vi "CHS_TRAJECTORY_EXECUTE_ABS.vi"(6 "Pass_Through_Time":dbl=-1.0 format="%33.4f", 8 "Init":bool, 11 "TrajectoryName":string) -> (1 "Complete":bool, 2 "AtReference":bool, 3 "Chassis Velocity Target SI":T1 {"vOmega" format="%10.3f"; "vY" format="%10.3f"; "vX" format="%10.3f"})   [LabVIEW 2019]
uses:
  CHS_TRAJECTORY_GLOBALS.vi
  <vilib>/Rock Robotics/WPI/ThirdParty/JAS_Junk/TrajLib/Trajectory_Library.lvlib
  <vilib>/Rock Robotics/WPI/ThirdParty/ChoreoLib/ChoreoLib.lvlib
  <vilib>/Rock Robotics/WPI/ThirdParty/JAS_Junk/TrajLib/TypeDef/CHASSIS_SPEEDS.ctl
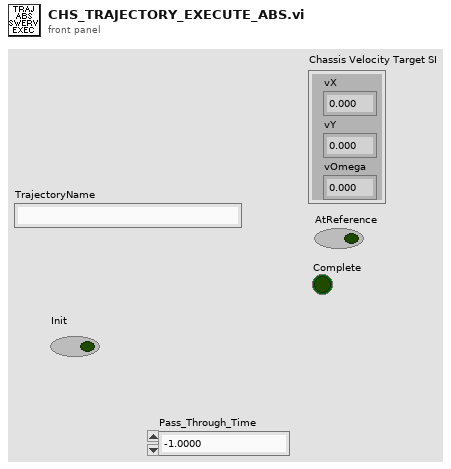
[diagram p1: front panel]
types:
  T1 = typedef "Trajectory_Library.lvlib/CHASSIS_SPEEDS.ctl" = cluster{"vX":dbl, "vY":dbl, "vOmega":dbl}
  T2 = typedef "Trajectory_Library.lvlib/PID_ADV_LIMITS.ctl" = cluster{"MaxInput":dbl, "MinInput":dbl, "Continuous":bool, "MaxOutput":dbl, "MinOutput":dbl}
  T3 = typedef "Trajectory_Library.lvlib/PID_ADV_TUNING.ctl" = cluster{"Kf":dbl, "Kp":dbl, "Ki":dbl, "Kd":dbl, "MaximumIntegral":dbl, "MinimumIntegral":dbl, "Filter Derivative":bool, "IntegralZone":dbl}
  T4 = typedef "Trajectory_Library.lvlib/POSE2D.ctl" = cluster{"TRANSLATION":T5, "ROTATION":T6}
  T5 = typedef "Trajectory_Library.lvlib/TRANSLATION2D.ctl" = cluster{"X":dbl, "Y":dbl}
  T6 = typedef "Trajectory_Library.lvlib/ROTATION2D.ctl" = cluster{"VALUE":dbl, "COS":dbl, "SIN":dbl}
  T7 = typedef "ChoreoLib.lvlib/ChoreoSwerveControlConfig.ctl" = cluster{"X_Adv PID Tuning":T3, "X_Adv PID Limits":T2, "Y_Adv PID Tuning":T3, "Y_Adv PID Limits":T2, "Rot_Adv PID Tuning":T3, "Rot_Adv PID Limits":T2, "X Y Pos Tolerance M":dbl, "Rot Tolerance Deg":dbl, "X Y Vel Tolerance M/S":dbl, "Rot Vel Tolerance Deg/S":dbl}
  T8 = cluster{"X Pos Err M":dbl, "X Vel Err M/S":dbl, "Y Pos Err M":dbl, "Y Vel Err M/S":dbl, "Rot Pos Err Deg":dbl, "Rot Vel Err Deg/Sec":dbl}
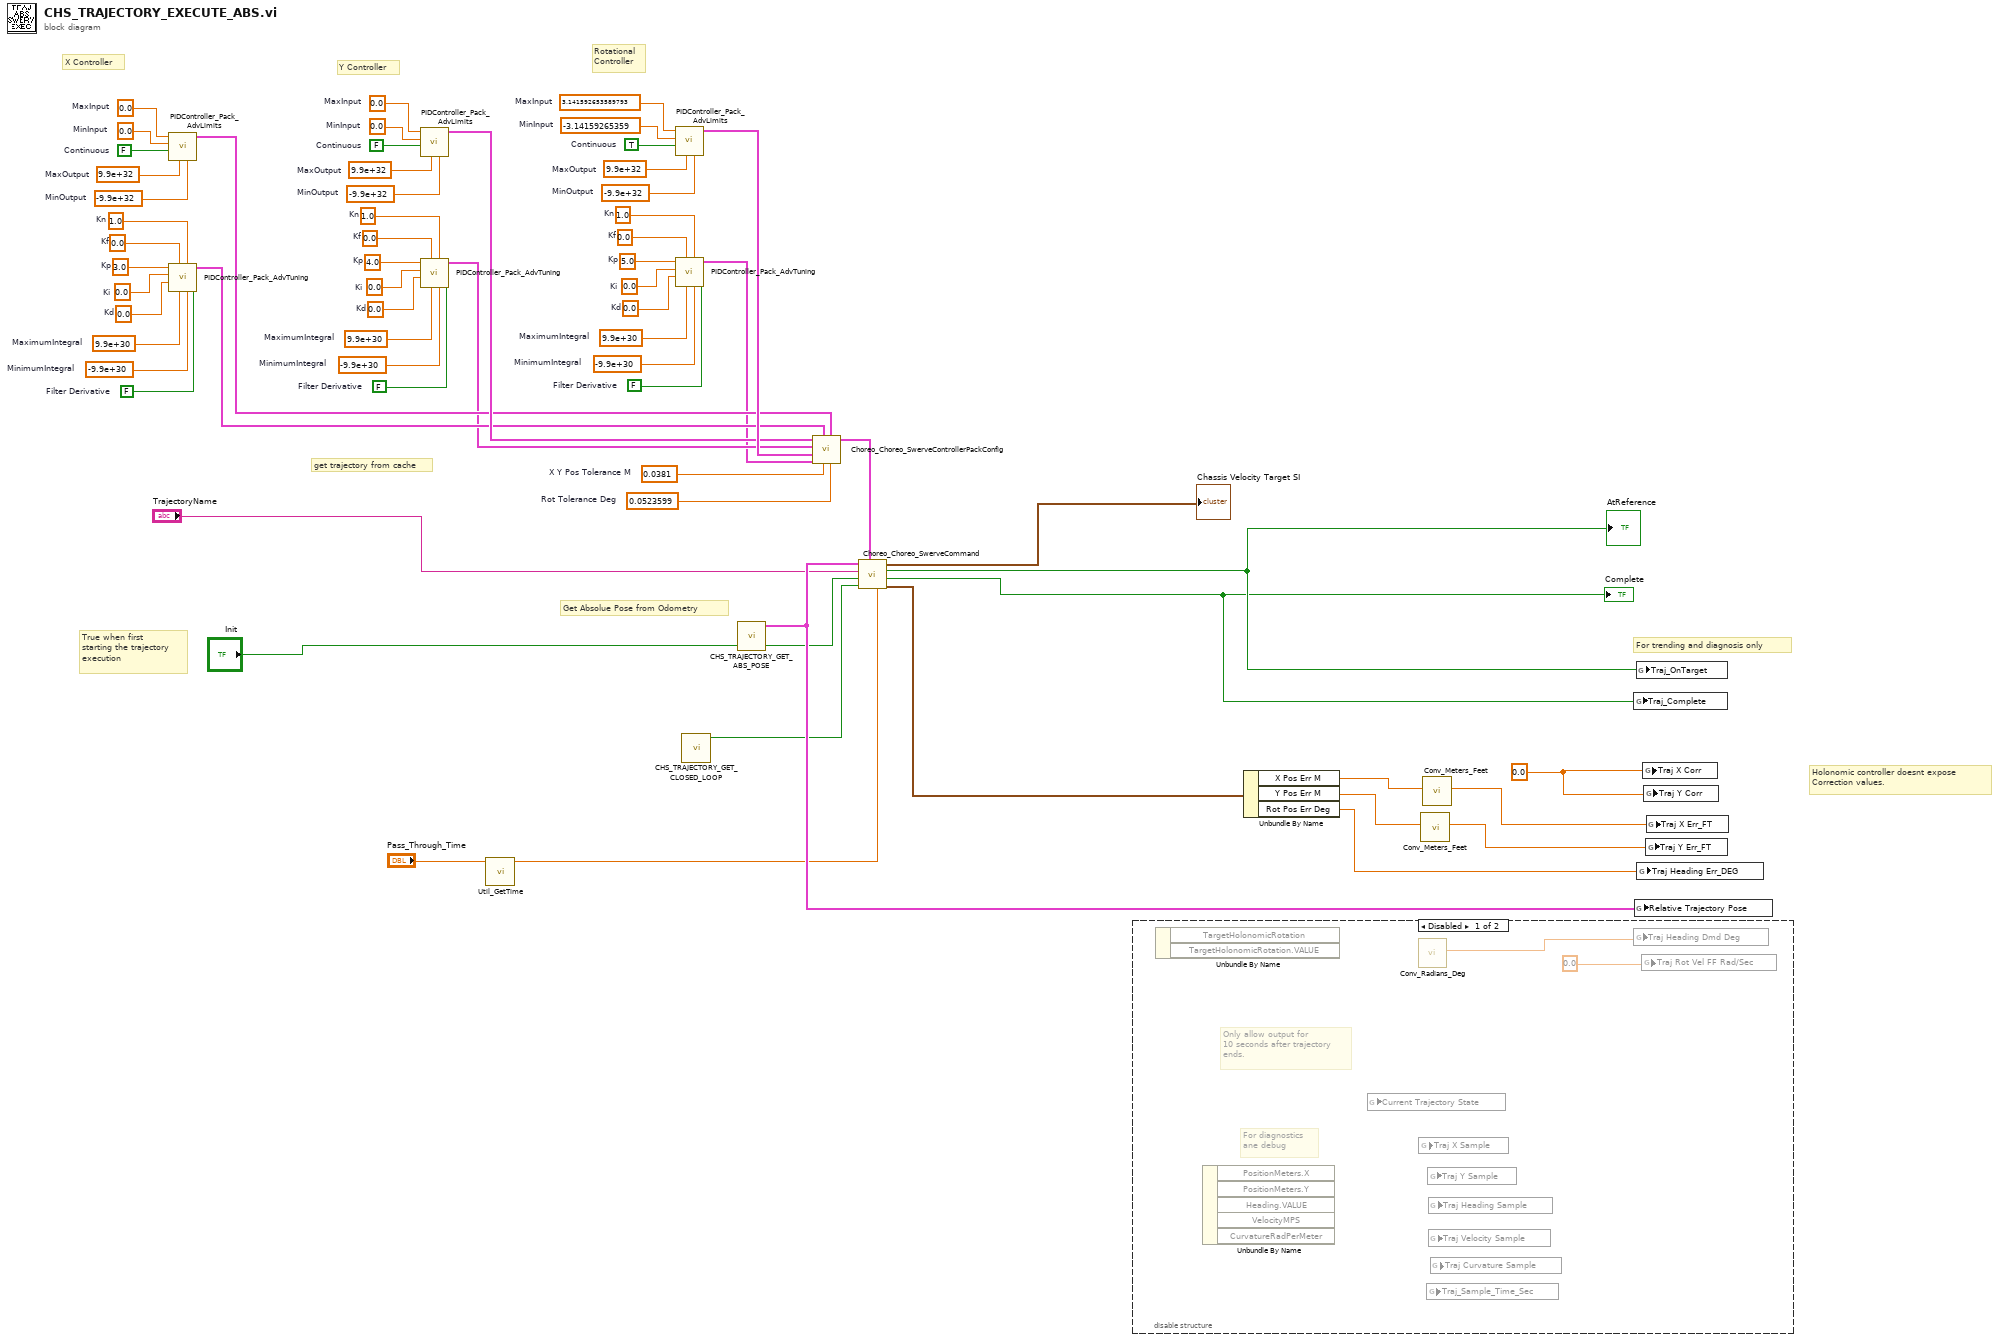
[diagram p0: block diagram]
diagram:
  w9 = 0.0 ("Y Corr")
  w64 = 0.0523599  # Rot Tolerance Deg
  w63 = 0.0381  # X Y Pos Tolerance M
  w44 = 1.0  # Kn
  w45 = 5.0  # Kp
  w46 = 0.0  # Ki
  w47 = 0.0  # Kd
  w48 = 0.0  # Kf
  w49 = 9.9e+30  # MaximumIntegral
  w50 = -9.9e+30  # MinimumIntegral
  w51 = FALSE  # Filter Derivative
  w53 = -3.14159265359  # MinInput
  w54 = TRUE  # Continuous
  w55 = 9.9e+32  # MaxOutput
  w52 = -9.9e+32  # MinOutput
  w56 = 3.141592653589793  # MaxInput
  w31 = 1.0  # Kn
  w32 = 4.0  # Kp
  w33 = 0.0  # Ki
  w34 = 0.0  # Kd
  w35 = 0.0  # Kf
  w36 = 9.9e+30  # MaximumIntegral
  w37 = -9.9e+30  # MinimumIntegral
  w38 = FALSE  # Filter Derivative
  w40 = 0.0  # MinInput
  w41 = FALSE  # Continuous
  w42 = 9.9e+32  # MaxOutput
  w39 = -9.9e+32  # MinOutput
  w43 = 0.0  # MaxInput
  w18 = 1.0  # Kn
  w19 = 3.0  # Kp
  w20 = 0.0  # Ki
  w21 = 0.0  # Kd
  w22 = 0.0  # Kf
  w23 = 9.9e+30  # MaximumIntegral
  w24 = -9.9e+30  # MinimumIntegral
  w25 = FALSE  # Filter Derivative
  w27 = 0.0  # MinInput
  w28 = FALSE  # Continuous
  w29 = 9.9e+32  # MaxOutput
  w26 = -9.9e+32  # MinOutput
  w30 = 0.0  # MaxInput
  # "get trajectory from cache"
  # "Rotational\nController"
  # "Y Controller"
  # "X Controller"
  # "True when first\nstarting the trajectory\nexecution"
  # "Holonomic controller doesnt expose\nCorrection values."
  # "For trending and diagnosis only"
  # "Get Absolue Pose from Odometry"
  n1 = call <vilib>:"PIDController_Pack_AdvLimits.vi"("MinOutput"=w26, "MaxOutput"=w29, "Continuous"=w28, "MinInput"=w27, "MaxInput"=w30) -> ("Adv PID Limits"=w60:T2)  [unwired: 6 in]
  n2 = call <vilib>:"PIDController_Pack_AdvTuning.vi"("Filter Derivative"=w25, "MinimumIntegral"=w24, "Kn"=w18, "MaximumIntegral"=w23, "Kf"=w22, "Kd"=w21, "Ki"=w20, "Kp"=w19) -> ("Adv PID Tuning"=w59:T3)  [unwired: 3 in]
  n3 = call <vilib>:"PIDController_Pack_AdvLimits.vi"("MinOutput"=w39, "MaxOutput"=w42, "Continuous"=w41, "MinInput"=w40, "MaxInput"=w43) -> ("Adv PID Limits"=w61:T2)  [unwired: 6 in]
  n4 = call <vilib>:"PIDController_Pack_AdvTuning.vi"("Filter Derivative"=w38, "MinimumIntegral"=w37, "Kn"=w31, "MaximumIntegral"=w36, "Kf"=w35, "Kd"=w34, "Ki"=w33, "Kp"=w32) -> ("Adv PID Tuning"=w58:T3)  [unwired: 3 in]
  n5 = call <vilib>:"Util_GetTime.vi"("Pass_Through_Time"="Pass_Through_Time") -> ("FPGA_Time_Seconds"=w10:dbl)  [unwired: 8 in, 2 out]
  n6 = call <vilib>:"PIDController_Pack_AdvLimits.vi"("MinOutput"=w52, "MaxOutput"=w55, "Continuous"=w54, "MinInput"=w53, "MaxInput"=w56) -> ("Adv PID Limits"=w62:T2)  [unwired: 6 in]
  n7 = call <vilib>:"PIDController_Pack_AdvTuning.vi"("Filter Derivative"=w51, "MinimumIntegral"=w50, "Kn"=w44, "MaximumIntegral"=w49, "Kf"=w48, "Kd"=w47, "Ki"=w46, "Kp"=w45) -> ("Adv PID Tuning"=w57:T3)  [unwired: 3 in]
  n8 = call "CHS_TRAJECTORY_GET_CLOSED_LOOP.vi"() -> ("AUTO_CLOSED_LOOP"=w15:bool)  [unwired: 11 in]
  n9 = call "CHS_TRAJECTORY_GET_ABS_POSE.vi"() -> ("Absolute Odometry Pose"=w16:T4)  [unwired: 11 in]
  n10 = call <vilib>:"Choreo_Choreo_SwerveControllerPackConfig.vi"("Rot Tolerance Deg"=w64, "X_Adv PID Limits"=w60, "X Y Pos Tolerance M"=w63, "X_Adv PID Tuning"=w59, "Rot_Adv PID Tuning"=w57, "Rot_Adv PID Limits"=w62, "Y_Adv PID Tuning"=w58, "Y_Adv PID Limits"=w61) -> ("ChoreoSwerveControlConfig"=w17:T7)  [unwired: 3 in]
  n11 = call <vilib>:"Choreo_Choreo_SwerveCommand.vi"("Pass_Through_Time"=w10, "ChoreoSwerveControlConfig"=w17, "Auto"=w15, "Initialize"="Init", "TrajectoryName"="TrajectoryName", "Current Position"=w16) -> ("Ctrl Info"=w6:T8, "Complete"=w12:bool, "On Target"=w13:bool, "Chassis Speed Dmd"=→"Chassis Velocity Target SI":T1)  [unwired: 2 in]
  "AtReference" <- w13
  "Complete" <- w12
  n12 = disable-structure shown="Disabled" {
    frame Disabled {
      # "For diagnostics\nane debug"
      # "Only allow output for\n10 seconds after trajectory\nends."
      n13 = Unbundle By Name() -> ()  [unwired: 1 in, 2 out]
      n14 = Unbundle By Name() -> ()  [unwired: 1 in, 5 out]
      n15 = global read "CHS_TRAJECTORY_GLOBALS.vi" "Current Trajectory State"() -> ()  [unwired: 1 in]
      n16 = call <vilib>:"Conv_Radians_Deg.vi"() -> ("Degrees"=w65:dbl)  [unwired: 11 in]
      n17 = global read "CHS_TRAJECTORY_GLOBALS.vi" "Traj X Sample"() -> ()  [unwired: 1 in]
      n18 = global read "CHS_TRAJECTORY_GLOBALS.vi" "Traj_Sample_Time_Sec"() -> ()  [unwired: 1 in]
      n19 = global read "CHS_TRAJECTORY_GLOBALS.vi" "Traj Y Sample"() -> ()  [unwired: 1 in]
      n20 = global read "CHS_TRAJECTORY_GLOBALS.vi" "Traj Heading Sample"() -> ()  [unwired: 1 in]
      n21 = global read "CHS_TRAJECTORY_GLOBALS.vi" "Traj Velocity Sample"() -> ()  [unwired: 1 in]
      n22 = global read "CHS_TRAJECTORY_GLOBALS.vi" "Traj Curvature Sample"() -> ()  [unwired: 1 in]
      n23 = global write "CHS_TRAJECTORY_GLOBALS.vi" "Traj Heading Dmd Deg"(w65) -> ()
      n24 = global write "CHS_TRAJECTORY_GLOBALS.vi" "Traj Rot Vel FF Rad/Sec"(0.0 ("Traj Heading Dmd Deg")) -> ()
    }
    frame Enabled {
    }
  }
  n25 = Unbundle By Name(w6) -> ("X Pos Err M"=w5:dbl, "Y Pos Err M"=w4:dbl, "Rot Pos Err Deg"=w3:dbl)
  n26 = call <vilib>:"Conv_Meters_Feet.vi"("Meters"=w4) -> ("Feet"=w8:dbl)  [unwired: 10 in]
  n27 = call <vilib>:"Conv_Meters_Feet.vi"("Meters"=w5) -> ("Feet"=w7:dbl)  [unwired: 10 in]
  n28 = global write "CHS_TRAJECTORY_GLOBALS.vi" "Traj_Complete"(w12) -> ()
  n29 = global write "CHS_TRAJECTORY_GLOBALS.vi" "Relative Trajectory Pose"(w16) -> ()
  n30 = global write "CHS_TRAJECTORY_GLOBALS.vi" "Traj_OnTarget"(w13) -> ()
  n31 = global write "CHS_TRAJECTORY_GLOBALS.vi" "Traj Heading Err_DEG"(w3) -> ()
  n32 = global write "CHS_TRAJECTORY_GLOBALS.vi" "Traj X Corr"(w9) -> ()
  n33 = global write "CHS_TRAJECTORY_GLOBALS.vi" "Traj Y Corr"(w9) -> ()
  n34 = global write "CHS_TRAJECTORY_GLOBALS.vi" "Traj Y Err_FT"(w8) -> ()
  n35 = global write "CHS_TRAJECTORY_GLOBALS.vi" "Traj X Err_FT"(w7) -> ()
